vi "CRYASIOGetOutputDeviceNames.vi"(10 "Driver Name":string, 11 "error in (no error)":errorcluster) -> (1 "Channel Idx":u32[](array[numeric]), 2 "Output Device Names":string[](array[string]), 3 "error out":errorcluster)   [LabVIEW 2013]
uses:
  CRY_ASIO.dll
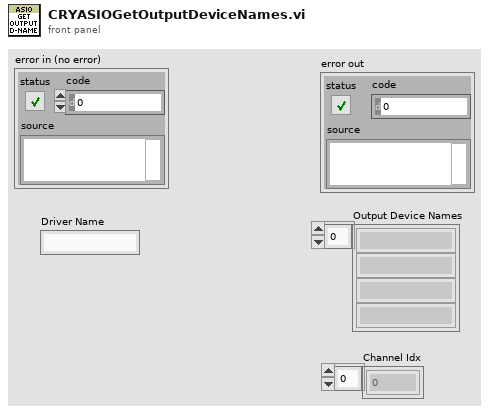
[diagram p1: front panel]
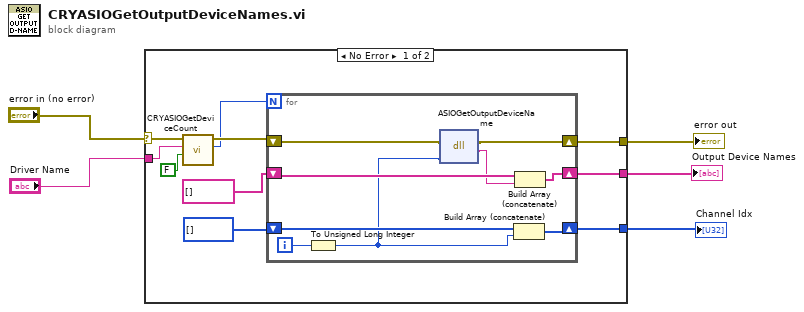
[diagram p0: block diagram]
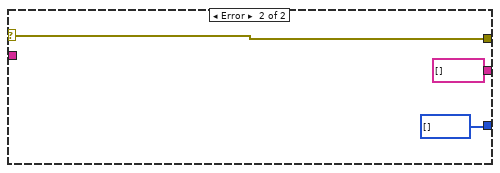
[diagram p2: hidden frame]
diagram:
  n1 = case shown="No Error" "error in (no error)" {
    selector: "error in (no error)" -> [w12 w26]
    tunnel: "Driver Name" -> [w9 _]
    tunnel: [w14 w26] -> w2
    tunnel: [w13 string[] [] ("appended array")] -> w3
    tunnel: [w6 i32[] [] ("appended array")] -> w1
    frame No Error {
      n2 = call "CRYASIOGetDeviceCount.vi"("InOut"=FALSE, "Driver Name"=w9, "error in (no error)"=w12) -> ("Device Count"=w10:u32, "error out"=w11:errorcluster)  [unwired: 7 in]
      n3 = for {
        N: w10 -> [_]
        shift-right: [w23] -> w13
        shift-left: string[] [] ("appended array") -> [w24]
        shift-right: [w20] -> w14
        shift-left: w11 -> [w21]
        shift-right: [w17] -> w6
        shift-left: i32[] [] ("appended array") -> [w18]
        i -> [w22]
        n4 = To Unsigned Long Integer(number=w22) -> (unsigned 32bit integer=w16:u32)
        n5 = dll-call lib="D:/LabView_Project/CRY6181/CRY_ASIO.dll" fn="ASIOGetOutputDeviceName"(error in=w21, "devID"=w16) -> (error out=w20:errorcluster, "return type"=w19:string)  [unwired: 3 in, 1 out]
        n6 = Build Array (concatenate)(w18, w16) -> (w17:u32[])
        n7 = Build Array (concatenate)(w24, w19) -> (w23:string[])
      }
    }
    frame Error {
    }
  }
  "Output Device Names" <- w3
  "error out" <- w2
  "Channel Idx" <- w1
